vi "DS_Write Wrapper.vi"(0 "Shared Variable":refnum<k21>, 2 "rawData":variant, 3 "ms timeout (0)":i32, 5 "error in":errorcluster) -> (17 "timed out":bool, 19 "error out":errorcluster)   [LabVIEW 2012, in "HGF_DSC.lvlib"]
uses:
  HGF_DSC.lvlib
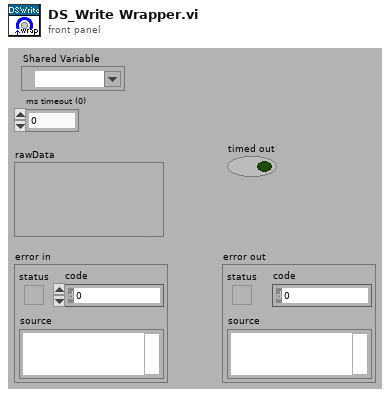
[diagram p1: front panel]
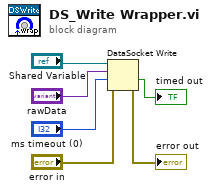
[diagram p0: block diagram]
diagram:
  n1 = DataSocket Write(8:"error in", 9:"ms timeout (0)", 10:"rawData", 11:"Shared Variable") -> (0:→"error out":errorcluster, 1:→"timed out":bool)  [unwired: 1 out]
